vi "Test.vi"(8 "error in (no error)":errorcluster, 11 "PostStep in":refnum<class "PostStep.lvclass">) -> (0 "error out":errorcluster, 2 "Pass?":bool, 3 "PostStep out":refnum<class "PostStep.lvclass">)   [LabVIEW 2020, in "PostStep.lvclass"]
uses:
  PostStep.lvclass
  Base Decorator/Base Decorator.lvclass
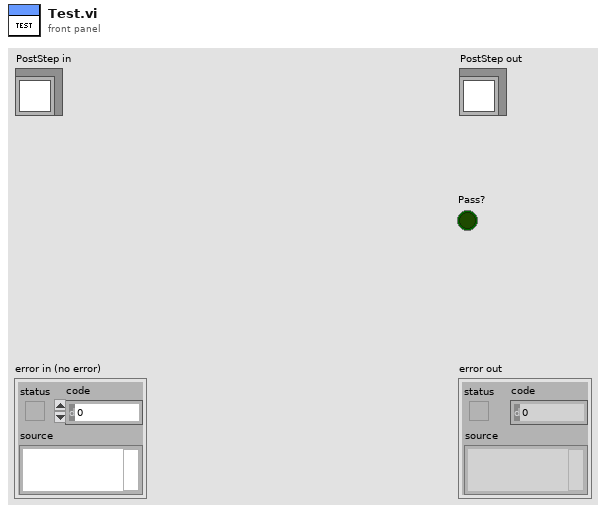
[diagram p1: front panel]
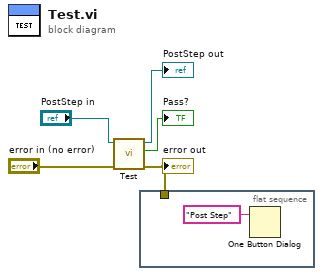
[diagram p0: block diagram]
diagram:
  n1 = call-parent "Test.vi"("error in (no error)"="error in (no error)", "Base Decorator in"="PostStep in") -> ("error out"=w1:errorcluster, "Pass?"=→"Pass?":bool, "Base Decorator out"=→"PostStep out":refnum<class "PostStep.lvclass">)  [unwired: 7 in]
  "error out" <- w1
  n2 = flat-sequence {
    tunnel: w1 -> [_]
    frame #0 {
      n3 = One Button Dialog(message="Post Step") -> ()  [unwired: 1 in, 1 out]
    }
  }
